vi "Add credit.vi"(8 "error in (no error)":errorcluster, 10 "Credito":dbl, 11 "UI Actor in":refnum<class "UI Actor.lvclass">) -> (0 "error out":errorcluster, 3 "UI Actor out":refnum<class "UI Actor.lvclass">)   [LabVIEW 2020, in "UI Actor.lvlib" / "UI Actor.lvclass"]
uses:
  UI Actor.lvclass
  UI Actor.lvclass/UI Actor.ctl
  Msg Messages/Update Msg Msg/Update Msg Msg.lvclass/Update Msg Msg.ctl
  <vilib>/ActorFramework/Message Enqueuer/Message Enqueuer.lvclass/Message Enqueuer.ctl
  <vilib>/ActorFramework/Message Enqueuer/Enqueue.vi
  Msg Messages/Update Msg Msg/Update Msg Msg.lvclass
  C:/Program Files (x86)/National Instruments/LabVIEW 2020/vi.lib/ActorFramework/Message/Message.lvclass
  <vilib>/ActorFramework/Message Priority Queue/Priority Enqueue.vi
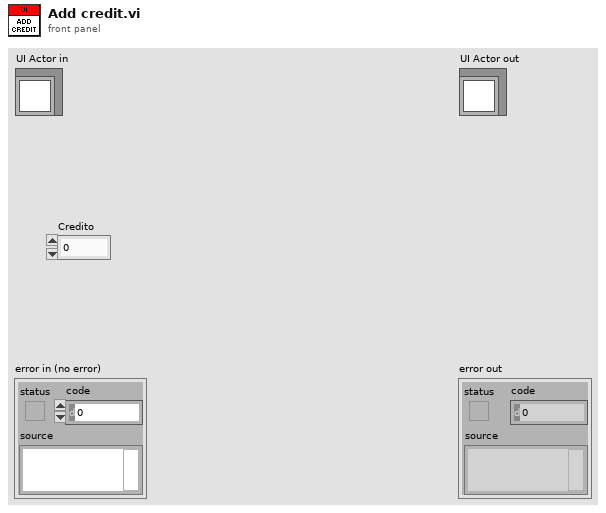
[diagram p1: front panel]
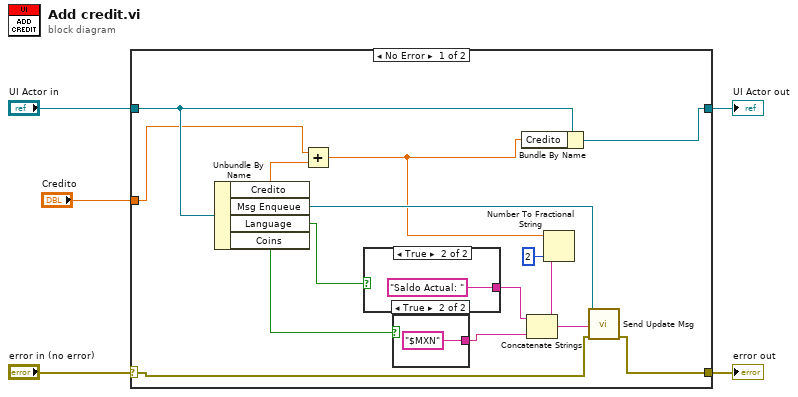
[diagram p0: block diagram]
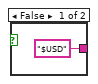
[diagram p2: hidden frame]
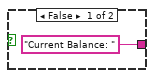
[diagram p3: hidden frame]
diagram:
  n1 = case shown="No Error" "error in (no error)" {
    selector: "error in (no error)" -> [w13 w26]
    tunnel: [w12 w26] -> w4
    tunnel: [w18 w25] -> w2
    tunnel: "UI Actor in" -> [w19 w25]
    tunnel: "Credito" -> [w10 _]
    frame No Error {
      n2 = Unbundle By Name(w19) -> ("Credito"=w9:dbl, "Msg Enqueue"=w20:refnum<class "Message Enqueuer.lvclass">, "Language"=w15:bool, "Coins"=w8:bool)
      n3 = Add(x=w10, y=w9) -> (x+y=w6:dbl)
      n4 = case shown="True" w15 {
        tunnel: ["Current Balance: " ("string") "Saldo Actual: " ("string")] -> w14
        frame False {
        }
        frame True {
        }
      }
      n5 = case shown="True" w8 {
        tunnel: ["$USD" ("string") "$MXN" ("string")] -> w7
        frame False {
        }
        frame True {
        }
      }
      n6 = Bundle By Name(cluster=w19, "Credito"=w6) -> (w18:refnum<class "UI Actor.lvclass">)
      n7 = Number To Fractional String(number=w6, precision (6)=i16 2) -> (F-format string=w17:string)  [unwired: 2 in]
      n8 = Concatenate Strings(w14, w17, w7) -> (w16:string)
      n9 = call "Send Update Msg.vi"("error in (no error)"=w13, "Update Msg"=w16, "Message Enqueuer"=w20) -> ("error out"=w12:errorcluster)  [unwired: 7 in, 1 out]
    }
    frame Error {
    }
  }
  "error out" <- w4
  "UI Actor out" <- w2
